vi "SendXML.vi"(2 "Send":string, 3 "URI in":string) -> (0 "error out":errorcluster, 1 "Reply":string)   [LabVIEW 2014]
doc: "Sends XML through a TCP network connection"
uses:
  <userlib>/ROS for LabVIEW Software.lnk/ROS/Code/_ROSDefinition.vi
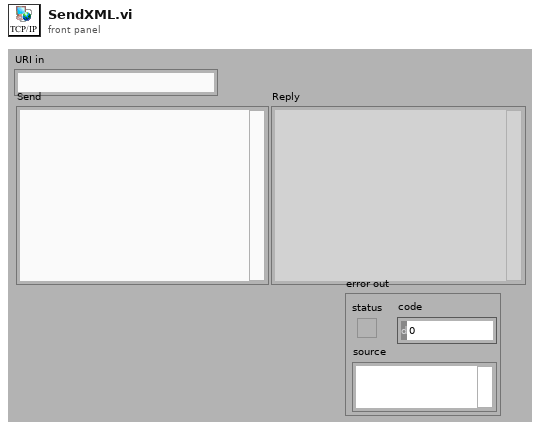
[diagram p1: front panel]
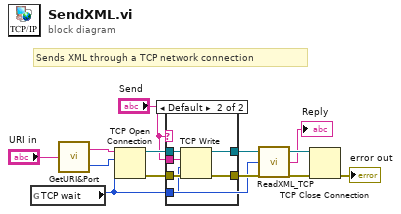
[diagram p0: block diagram]
diagram:
  # "Sends XML through a TCP network connection"
  n1 = global read "_ROSDefinition.vi" "TCP wait"() -> (w1:i32)
  n2 = call <userlib>:"GetURI&Port.vi"("URI in"="URI in") -> ("Port"=w13:u16, "URI"=w12:string)
  n3 = TCP Open Connection(address=w12, remote port or service name=w13, timeout ms (60000)=w1) -> (connection ID=w10:refnum<k5>, error out=w11:errorcluster)  [unwired: 2 in]
  n4 = case shown="Default" "Send" {
    tunnel: w11 -> [w14 w21]
    tunnel: w10 -> [w15 w20]
    tunnel: [w15 w19] -> w9
    tunnel: [w14 w18] -> w8
    tunnel: "Send" -> [_ w17]
    tunnel: w1 -> [_ w16]
    frame "" {
    }
    frame Default {
      n5 = TCP Write(connection ID=w20, data in=w17, error in (no error)=w21, 9:w16) -> (connection ID out=w19:refnum<k5>, error out=w18:errorcluster)  [unwired: 1 out]
    }
  }
  n6 = call <userlib>:"ReadXML_TCP.vi"("error in"=w8, "timeout ms (3000)"=w1, "connection ID in"=w9) -> ("error out"=w6:errorcluster, "data out"=→"Reply":string, "connection ID out"=w5:refnum<k5>)
  n7 = TCP Close Connection(connection ID=w5, error in (no error)=w6) -> (error out=→"error out":errorcluster)  [unwired: 1 in, 1 out]
